vi "Read Rx Command.vi"(8 "error in (no error)":errorcluster, 11 "RxTx in":refnum<class "CCS_RxTx.lvclass">) -> (0 "error out":errorcluster, 2 "Rx Command":string, 3 "RxTx out":refnum<class "CCS_RxTx.lvclass">)   [LabVIEW 2018, in "CCS_RxTx.lvclass"]
uses:
  CCS_RxTx.lvclass
  CCS_RxTx.lvclass/CCS_RxTx.ctl
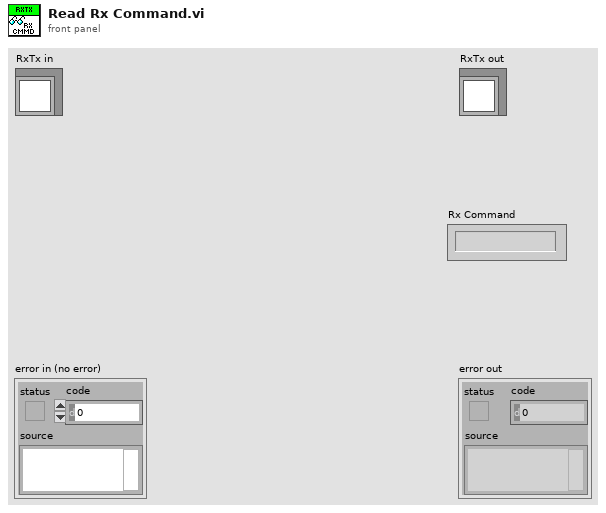
[diagram p1: front panel]
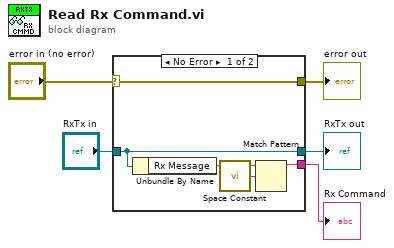
[diagram p0: block diagram]
diagram:
  n1 = case shown="No Error" "error in (no error)" {
    selector: "error in (no error)" -> [w10 w12]
    tunnel: [w10 w12] -> w4
    tunnel: [w9 w11] -> w2
    tunnel: "RxTx in" -> [w9 w11]
    tunnel: [w6 _] -> w1
    frame No Error {
      n2 = Unbundle By Name(w9) -> ("Rx Message"=w8:string)
      n3 = call <vilib>:"Space Constant.vi"() -> ("String"=w7:string)
      n4 = Match Pattern(string=w8, regular expression=w7) -> (before substring=w6:string)  [unwired: 1 in, 3 out]
    }
    frame Error {
    }
  }
  "error out" <- w4
  "RxTx out" <- w2
  "Rx Command" <- w1
